vi "Uncompress Digital.vi"   [LabVIEW 2011]
doc: "Uncompresses the digital signals in the digital input and returns the result in the digital output. Wire data to the <B>uncompressed digital waveform</B> input to determine the polymorphic instance to use or manually select the instance."
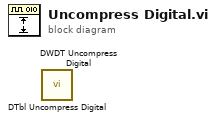
[diagram p0: block diagram]
diagram:
  n1 = call "DTbl Uncompress Digital.vi"() -> ()  [unwired: 10 in, 2 out]
  n2 = call "DWDT Uncompress Digital.vi"() -> ()  [unwired: 10 in, 2 out]
